vi "mod_Pilot tone filter design.vi"(0 "pilot extraction filter":T2={"taps"=81, "approx freq. (Hz)"=0.0, "search (+/- % of Fsampl) "=0.25}, 5 "sampling frequency":dbl, 11 "error in (no error)":errorcluster, 13 "reset? (T)":bool=TRUE) -> (4 "pilot extraction filter coefficients":dbl[](array[numeric]), 6 "pilot rejection filter coefficients":dbl[](array[numeric]), 8 "filter information":T1 {"Pilot rejection filter"."df" format="%.2p"; "Pilot rejection filter"."f0" format="%.2p"; "Pilot rejection filter"."Mag H(w)" format="%.2p"; "Pilot extraction filter"."df" format="%.2p"; "Pilot extraction filter"."f0" format="%.2p"; "Pilot extraction filter"."Mag H(w)" format="%.2p"}, 15 "error out":errorcluster)   [LabVIEW 2020, in "niAMT.lvlib"]
uses:
  <vilib>/addons/Modulation/niAMT.lvlib
  <vilib>/addons/Modulation/Analog/controls/mod_AM pilot extraction filter.ctl
  <vilib>/addons/Modulation/Analog/controls/mod_AM pilot filter info.ctl
  <vilib>/measure/maspectr.llb/FFT Spectrum (Mag-Phase) for 1 Chan.vi
  <vilib>/measure/NI_MAPro.lvlib
  <vilib>/Analysis/NI_AALBase.lvlib
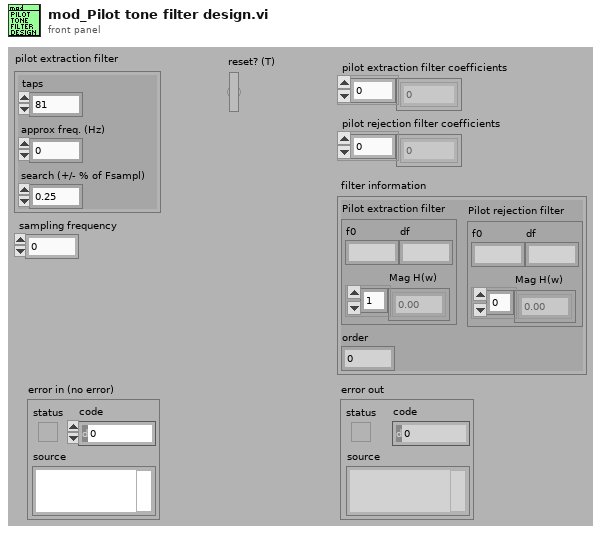
[diagram p1: front panel]
types:
  T1 = typedef "niAMT.lvlib/mod_AM pilot filter info.ctl" = cluster{"Pilot extraction filter":cluster{"f0":dbl, "df":dbl, "Mag H(w)":dbl[]}, "order":i32, "Pilot rejection filter":cluster{"f0":dbl, "df":dbl, "Mag H(w)":dbl[]}}
  T2 = typedef "niAMT.lvlib/mod_AM pilot extraction filter.ctl" = cluster{"taps":i32, "approx freq. (Hz)":dbl, "search (+/- % of Fsampl) ":dbl}
  T3 = cluster{"dB On (F)":bool, "unwrap phase (F)":bool, "convert to degree (F)":bool}
  T4 = enum32{"None", "Hanning", "Hamming", "Triangular", "Blackman", "Exact Blackman", "Blackman-Harris", "Kaiser-Bessel", "Flat Top"}
  T5 = enum32{"Lowpass", "Highpass", "Bandpass", "Bandstop"}
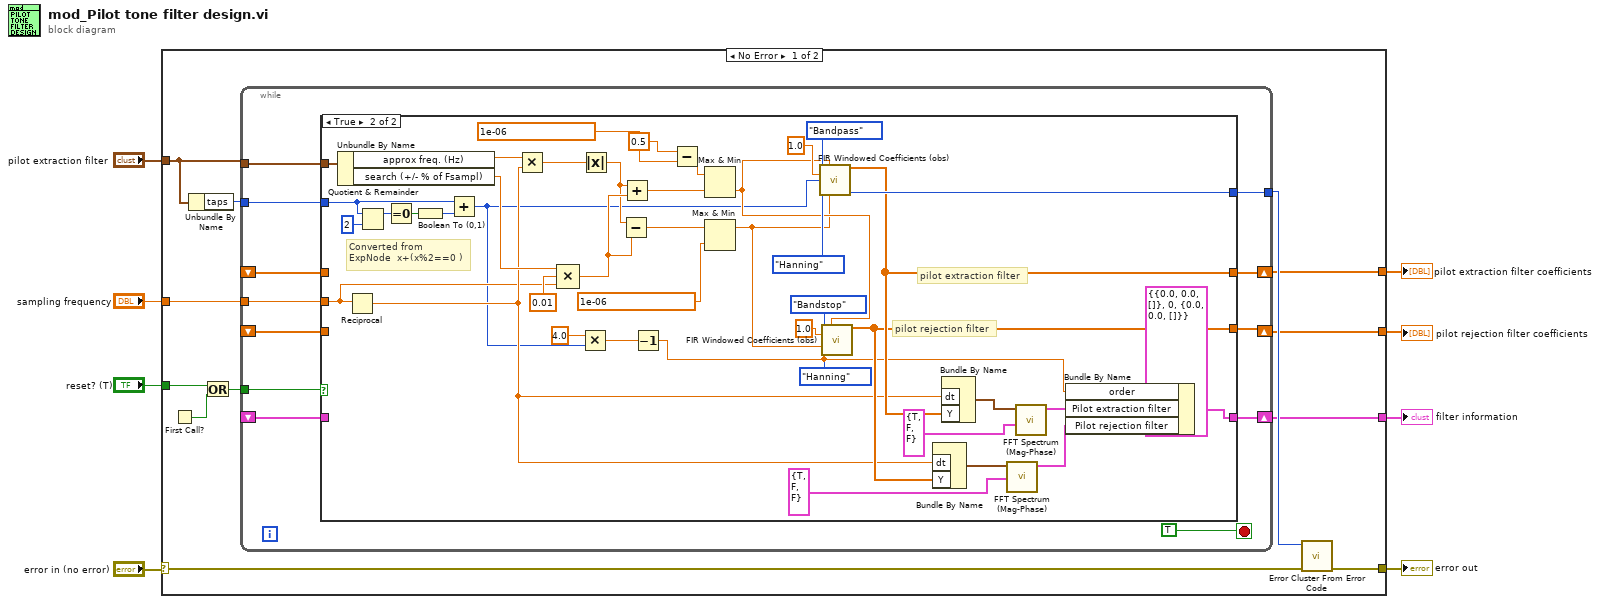
[diagram p0: block diagram]
diagram:
  n1 = case shown="No Error" "error in (no error)" {
    selector: "error in (no error)" -> [w13 w79]
    tunnel: "pilot extraction filter" -> [w17 _]
    tunnel: "reset? (T)" -> [w16 _]
    tunnel: [w14 w79] -> w5
    tunnel: [w12 _] -> w3
    tunnel: [w11 _] -> w4
    tunnel: "sampling frequency" -> [w10 _]
    tunnel: [w9 _] -> w1
    frame No Error {
      n2 = First Call?() -> (First Call?: T/F=w19:bool)
      n3 = Unbundle By Name(w17) -> ("taps"=w20:i32)
      n4 = Or(x=w16, y=w19) -> (x .or. y?=w18:bool)
      n5 = while {
        tunnel: w17 -> [w32]
        shift-right: [w30] -> w12
        shift-left: _ -> [w29]
        tunnel: [w28] -> w15
        tunnel: w20 -> [w27]
        tunnel: w18 -> [w26]
        shift-right: [w25] -> w11
        shift-left: _ -> [w24]
        tunnel: w10 -> [w23]
        shift-right: [w22] -> w9
        shift-left: _ -> [w21]
        stop <- TRUE stop-if-true
        n6 = case shown="True" w26 {
          tunnel: w32 -> [_ w73]
          tunnel: [w35 w56] -> w30
          tunnel: w29 -> [w35 _]
          tunnel: [_ w72] -> w28
          tunnel: w27 -> [_ w37]
          tunnel: [w34 w55] -> w25
          tunnel: w24 -> [w34 _]
          tunnel: w23 -> [_ w45]
          tunnel: [w33 w47] -> w22
          tunnel: w21 -> [w33 _]
          frame False {
          }
          frame True {
            # "Converted from\nExpNode \tx+(x%2==0 )"
            # "pilot rejection filter"
            # "pilot extraction filter"
            n7 = Unbundle By Name(w73) -> ("approx freq. (Hz)"=w63:dbl, "search (+/- % of Fsampl)"=w76:dbl)
            n8 = Reciprocal(x=w45) -> (1/x=w46:dbl)
            n9 = Quotient & Remainder(x=w37, y=2) -> (x-y*floor(x/y)=w40:i32)  [unwired: 1 out]
            n10 = Equal To 0?(x=w40) -> (x = 0?=w39:bool)
            n11 = Boolean To (0,1)(Boolean=w39) -> (0, 1=w41:i16)
            n12 = Add(x=w37, y=w41) -> (x+y=w36:i32)
            n13 = Multiply(x=w63, y=w46) -> (x*y=w57:dbl)
            n14 = Compound Arithmetic op=MULTIPLY(w76, 0.01, w45) -> (w75:dbl)
            n15 = Multiply(x=4.0, y=w36) -> (x*y=w44:dbl)
            n16 = Absolute Value(x=w57) -> (abs(x)=w64:dbl)
            n17 = Subtract(x=w64, y=w75) -> (x-y=w70:dbl)
            n18 = Add(x=w64, y=w75) -> (x+y=w69:dbl)
            n19 = Decrement(x=w44) -> (x-1=w42:dbl)
            n20 = Subtract(x=0.5, y=1e-06) -> (x-y=w66:dbl)
            n21 = Max & Min(x=w66, y=w69) -> (min(x,y)=w59:dbl)  [unwired: 1 out]
            n22 = Max & Min(x=w70, y=1e-06) -> (max(x,y)=w58:dbl)  [unwired: 1 out]
            n23 = call <vilib>:"FIR Windowed Coefficients (obs).vi"("filter type"=T5."Bandpass", "high cutoff freq: fh"=w59, "sampling freq: fs"=1.0, "taps"=w36, "window"=T4."Hanning", "low cutoff freq: fl"=w58) -> ("FIR Windowed Coefficients"=w56:dbl[], "error"=w72:i32)  [unwired: 1 in, 7 out]
            n24 = call <vilib>:"FIR Windowed Coefficients (obs).vi"("filter type"=T5."Bandstop", "high cutoff freq: fh"=w59, "sampling freq: fs"=1.0, "taps"=w42, "window"=T4."Hanning", "low cutoff freq: fl"=w58) -> ("FIR Windowed Coefficients"=w55:dbl[])  [unwired: 1 in, 8 out]
            n25 = Bundle By Name("dt"=w46, "Y"=w55) -> (w54:waveform(dbl))  [unwired: 1 out]
            n26 = Bundle By Name("dt"=w46, "Y"=w56) -> (w53:waveform(dbl))  [unwired: 1 out]
            n27 = call-poly <vilib>:"FFT Spectrum (Mag-Phase).vi"("view"=T3 {"dB On (F)"=TRUE, "unwrap phase (F)"=FALSE, "convert to degree (F)"=FALSE}, "time signal"=w54) -> ("magnitude"=w49:cluster{"f0":dbl, "df":dbl, "magnitude":dbl[]})  [unwired: 5 in, 4 out]
            n28 = call-poly <vilib>:"FFT Spectrum (Mag-Phase).vi"("view"=T3 {"dB On (F)"=TRUE, "unwrap phase (F)"=FALSE, "convert to degree (F)"=FALSE}, "time signal"=w53) -> ("magnitude"=w50:cluster{"f0":dbl, "df":dbl, "magnitude":dbl[]})  [unwired: 5 in, 4 out]
            n29 = Bundle By Name(cluster=T1 {"Pilot extraction filter"={"f0"=0.0, "df"=0.0, "Mag H(w)"=[]}, "order"=0, "Pilot rejection filter"={"f0"=0.0, "df"=0.0, "Mag H(w)"=[]}} ("filter information"), "order"=w42, "Pilot extraction filter"=w50, "Pilot rejection filter"=w49) -> (w47:T1)
          }
        }
      }
      n30 = call <vilib>:"Error Cluster From Error Code.vi"("error in (no error)"=w13, "error code (0)"=w15) -> ("error out"=w14:errorcluster)  [unwired: 1 in, 6 out]
    }
    frame Error {
    }
  }
  "error out" <- w5
  "pilot extraction filter coefficients" <- w3
  "pilot rejection filter coefficients" <- w4
  "filter information" <- w1
